vi "fgt set sensor Custom Scale.vi"(8 "error in (no error)":errorcluster, 10 "Custom Scale":T1, 11 "sensorIndex":u32) -> (0 "error out":errorcluster)   [LabVIEW 2017, in "fgt_SDK.lvlib"]
doc: "Apply a custom scale factor on sensor read value. This function is useful in order to adapt read sensor value to physical measurement.\nFor example if a flow-unit is used with a special oil and it's calibration table is set to H2O, read flowrate is not correct.\nScale factor is applied using following formula: scaled_value = a*sensor_value + b*sensor_value^2 + c*sensor_value^3\nNote that this scale is also used for the regulation. Not supported by IPS."
uses:
  fgt_SDK.lvlib
  TypeDefs/fgt_SCALE.ctl
  dlls/fgt_SDK_32.dll
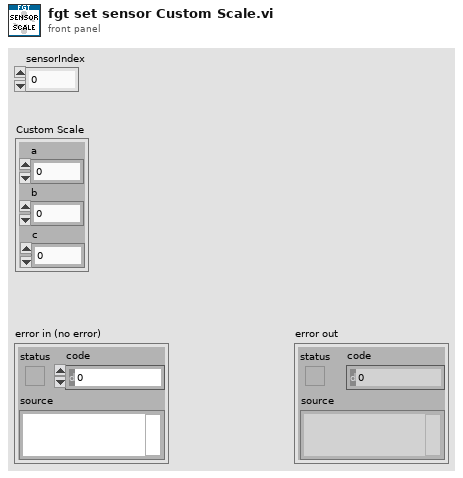
[diagram p1: front panel]
types:
  T1 = typedef "fgt_SDK.lvlib/fgt_SCALE.ctl" = cluster{"a":sgl, "b":sgl, "c":sgl}
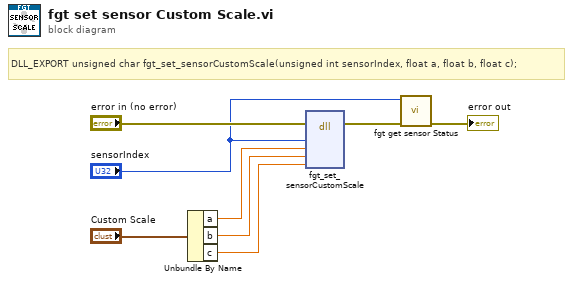
[diagram p0: block diagram]
diagram:
  # "DLL_EXPORT unsigned char fgt_set_sensorCustomScale(unsigned int sensorIndex, float a, float b, float c);"
  n1 = Unbundle By Name("Custom Scale") -> ("a"=w3:sgl, "b"=w2:sgl, "c"=w1:sgl)
  n2 = dll-call lib="D:/Work/SDK git/fgt-sdk-labview/dlls/fgt_SDK_*.*" fn="fgt_set_sensorCustomScale"(error in="error in (no error)", "sensorIndex"="sensorIndex", "a"=w3, "b"=w2, "c"=w1) -> (error out=w7:errorcluster)  [unwired: 7 in, 1 out]
  n3 = call "fgt get sensor Status.vi"("error in (no error)"=w7, "pressureIndex"="sensorIndex") -> ("error out"=→"error out":errorcluster)  [unwired: 9 in]
